vi "Test Notifiers.vi"   [LabVIEW 2019, in "Inst.Transport.lvclass"]
uses:
  Inst.Transport.lvclass
  Transport/Transport.lvclass
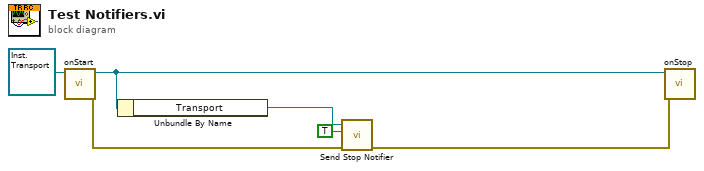
[diagram p0: block diagram]
diagram:
  n1 = call-dynamic "onStart.vi"("Inst.Transport"=refnum<class "Inst.Transport.lvclass"> refnum) -> ("error out"=w3:errorcluster, "Inst.Transport out"=w4:refnum<class "Inst.Transport.lvclass">)  [unwired: 9 in]
  n2 = Unbundle By Name(w4) -> ("Transport"=w5:refnum<class "Transport.lvclass">)
  n3 = call "Send Stop Notifier.vi"("error in (no error)"=w3, "Stop [T]"=TRUE, "Transport in"=w5) -> ("error out"=w2:errorcluster)  [unwired: 7 in, 1 out]
  n4 = call-dynamic "onStop.vi"("error in (no error)"=w2, "Inst.Transport"=w4) -> ()  [unwired: 8 in, 2 out]
